vi "Configure_AI_Module.vi"(8 "error in (no error)":errorcluster, 10 "AI_Module_Data":T1 {"Module_Data"."Address" format="%x"}, 11 "USB-87Pn":refnum<class "USB-87Pn.lvclass">) -> (0 "error out":errorcluster, 3 "USB-87Pn":refnum<class "USB-87Pn.lvclass">)   [LabVIEW 2019, in "USB-87Pn.lvlib" / "USB-87Pn.lvclass"]
uses:
  USB-87Pn.lvclass
  Module/AI_Module_Data.ctl
  Module/Module_Data.ctl
  USB-87Pn.lvclass/USB-87Pn.ctl
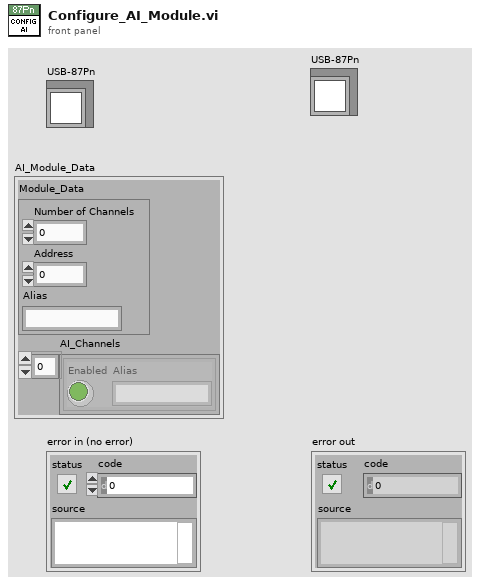
[diagram p1: front panel]
types:
  T1 = typedef "USB-87Pn.lvlib/USB-87Pn.lvclass/AI_Module_Data.ctl" = cluster{"Module_Data":T2, "AI_Channels":cluster{"Enabled":bool, "Alias":string}[]}
  T2 = typedef "USB-87Pn.lvlib/USB-87Pn.lvclass/Module_Data.ctl" = cluster{"Number of Channels":u8, "Address":i16, "Alias":string}
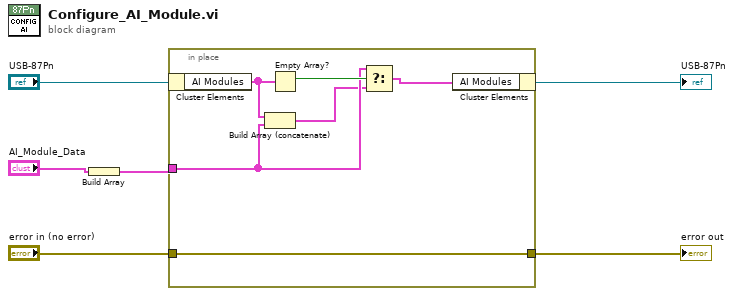
[diagram p0: block diagram]
diagram:
  n1 = Build Array("AI_Module_Data") -> (w1:T1[])
  n2 = in-place {
    in-place-border: "error in (no error)" -> [w12]
    in-place-border: w1 -> [w9]
    in-place-border: [w12] -> w3
    n3 = in-place-cluster #1("USB-87Pn") -> ("AI Modules"=w10:T1[])
    n4 = Build Array (concatenate)(w10, w9) -> (w8:T1[])
    n5 = Empty Array?(array=w10) -> (empty?=w11:bool)
    n6 = Select(t=w9, s=w11, f=w8) -> (s? t:f=w7:T1[])
    n7 = in-place-cluster #1("AI Modules"=w7) -> (→"USB-87Pn":refnum<class "USB-87Pn.lvclass">)
  }
  "error out" <- w3
